vi "clear_selection_list.vi"(6 "wait for reply (T)":bool=TRUE, 8 "error in":errorcluster, 11 "vi_id":i32) -> (0 "error out":errorcluster, 1 "timed out?":bool)   [LabVIEW 2025, in "Scripting Server.lvlib"]
doc: "Clears all elements in the selection list. Use this before making a new selection.\n\n_____\nCreated using DQMH Framework: Event Scripter 7.1.0.1503."
uses:
  Scripting Server.lvlib
  clear_selection_list Argument--cluster.ctl
  clear_selection_list (Reply Payload)--cluster.ctl
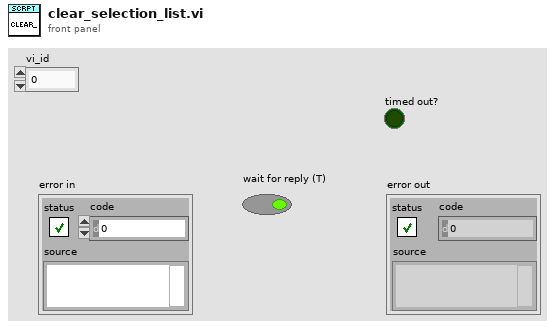
[diagram p1: front panel]
types:
  T1 = typedef "Scripting Server.lvlib/clear_selection_list Argument--cluster.ctl" = cluster{"Wait Notifier":refnum<notifier>, "wait for reply":bool, "vi_id":i32}
  T2 = typedef "Scripting Server.lvlib/Request Events--cluster.ctl" = cluster{"Stop Module":refnum<user-event>, "Show Panel":refnum<user-event>, "Hide Panel":refnum<user-event>, "Get Module Execution Status":refnum<user-event>, "Show Diagram":refnum<user-event>, "New VI":refnum<user-event>, "Add Object":refnum<user-event>, "Connect Objects":refnum<user-event>, "Get Object Terminals":refnum<user-event>, "get vi error list":refnum<user-event>, "Cleanup VI":refnum<user-event>, "create_control":refnum<user-event>, "Run VI":refnum<user-event>, "add_to_selection":refnum<user-event>, "clear_selection_list":refnum<user-event>, "remove_from_selection":refnum<user-event>, "enclose_selection":refnum<user-event>}
  T3 = typedef "Scripting Server.lvlib/clear_selection_list (Reply Payload)--cluster.ctl" = cluster{"error":errorcluster}
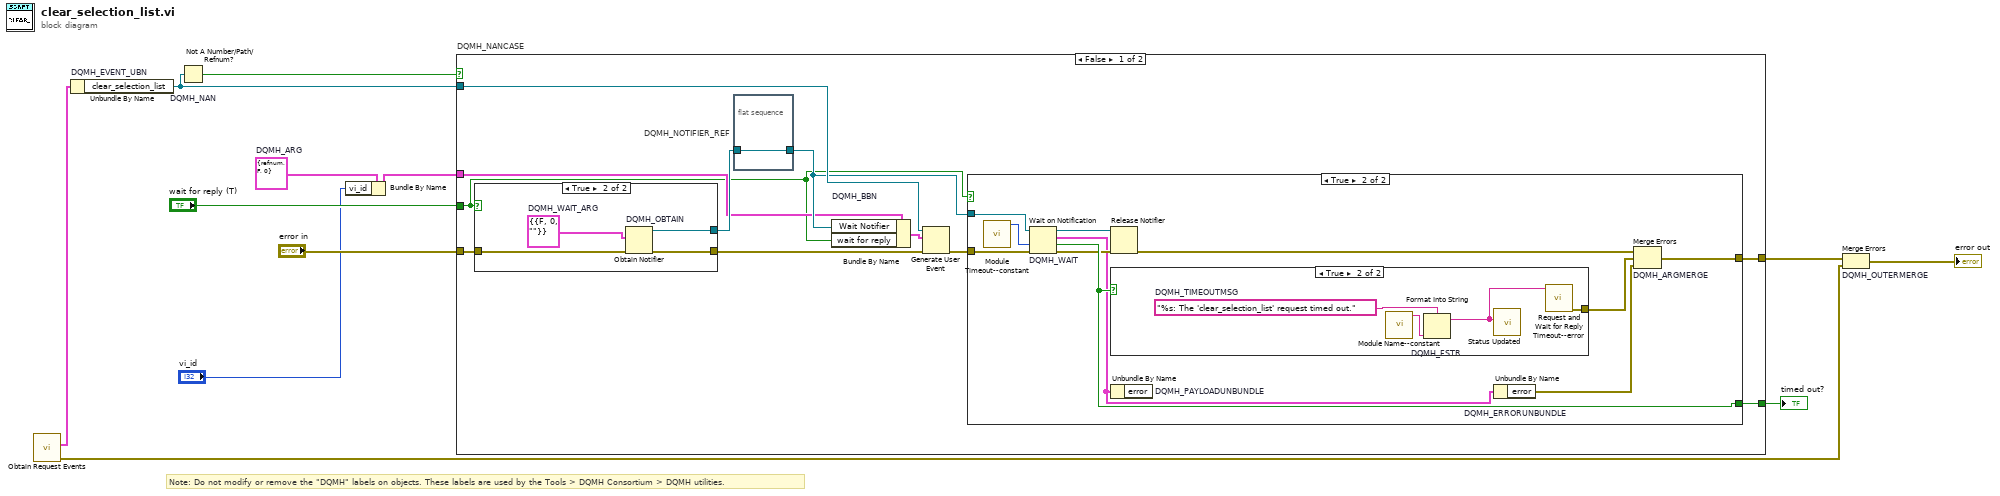
[diagram p0: block diagram]
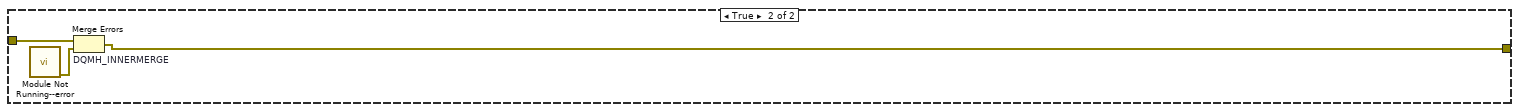
[diagram p5: hidden frame]
diagram:
  w6 = T1 {"Wait Notifier"=refnum, "wait for reply"=FALSE, "vi_id"=0}  # DQMH_ARG
  # "Note: Do not modify or remove the \"DQMH\" labels on objects. These labels are used by the Tools > DQMH Consortium > DQMH utilities."
  n1 = call "Obtain Request Events.vi"() -> ("error out"=w4:errorcluster, "Scripting Server Request Events"=w3:T2)  [unwired: 10 in]
  n2 = Unbundle By Name "DQMH_EVENT_UBN"(w3) -> ("clear_selection_list"=w10:refnum<user-event>)
  n3 = Not A Number/Path/Refnum? "DQMH_NAN"(number/path/refnum=w10) -> (NaN/Path/Refnum?=w9:bool)
  n4 = Bundle By Name(cluster=w6, "vi_id"="vi_id") -> (w2:T1)
  n5 = case "DQMH_NANCASE" shown="False" w9 {
    tunnel: "error in" -> [w23 w48]
    tunnel: w10 -> [w21 _]
    tunnel: [w18 w47] -> w7
    tunnel: [w19 _] -> w8
    tunnel: w2 -> [w14 _]
    tunnel: "wait for reply (T)" -> [w13 _]
    frame False {
      n6 = case shown="True" w13 {
        tunnel: w23 -> [w41 w45]
        tunnel: [w41 w44] -> w20
        tunnel: [_ w42] -> w16
        frame False {
        }
        frame True {
          w43 = T3 {"error"={"status"=FALSE, "code"=0, "source"=""}}  # DQMH_WAIT_ARG
          n7 = Obtain Notifier "DQMH_OBTAIN"(notification data type=w43, error in (no error)=w45) -> (notifier out=w42:refnum<notifier>, error out=w44:errorcluster)  [unwired: 2 in, 1 out]
        }
      }
      n8 = flat-sequence "DQMH_NOTIFIER_REF" {
        tunnel: w16 -> [w24]
        tunnel: [w24] -> w15
        frame #0 {
        }
      }
      n9 = Bundle By Name "DQMH_BBN"(cluster=w14, "Wait Notifier"=w15, "wait for reply"=w13) -> (w17:T1)
      n10 = Generate User Event(user event=w21, event data cluster=w17, error in=w20) -> (error out=w22:errorcluster)  [unwired: 1 in, 1 out]
      n11 = case shown="True" w13 {
        tunnel: w22 -> [w25 w36]
        tunnel: w15 -> [_ w35]
        tunnel: [_ w33] -> w19
        tunnel: [w25 w32] -> w18
        frame False {
        }
        frame True {
          n12 = call "Module Timeout--constant.vi"() -> ("Module Timeout"=w26:i32)  [unwired: 11 in]
          n13 = Wait on Notification "DQMH_WAIT"(notifier=w35, timeout in ms (-1)=w26, error in (no error)=w36) -> (notifier out=w34:refnum<notifier>, notification=w27:T3, timed out?=w33:bool, error out=w31:errorcluster)  [unwired: 1 in]
          n14 = Release Notifier(notifier=w34, error in (no error)=w31) -> (error out=w30:errorcluster)  [unwired: 1 in, 2 out]
          n15 = case shown="True" w33 {
            tunnel: [_ w38] -> w28
            frame False {
            }
            frame True {
              w40 = "%s: The 'clear_selection_list' request timed out."  # DQMH_TIMEOUTMSG
              n16 = call "Module Name--constant.vi"() -> ("Module Name"=w37:string)  [unwired: 11 in]
              n17 = Format Into String "DQMH_FSTR"(format string=w40, w37) -> (resulting string=w39:string)  [unwired: 2 in, 1 out]
              n18 = call "Status Updated.vi"("Status"=w39) -> ()  [unwired: 10 in, 1 out]
              n19 = call "Request and Wait for Reply Timeout--error.vi"("Error Message"=w39) -> ("error out"=w38:errorcluster)  [unwired: 10 in]
            }
          }
          n20 = Unbundle By Name "DQMH_PAYLOADUNBUNDLE"(w27) -> ()  [unwired: 1 out]
          n21 = Unbundle By Name "DQMH_ERRORUNBUNDLE"(w27) -> ("error"=w29:errorcluster)
          n22 = Merge Errors "DQMH_ARGMERGE"(w30, w28, w29) -> (w32:errorcluster)
        }
      }
    }
    frame True {
      n23 = call "Module Not Running--error.vi"() -> ("error out"=w46:errorcluster)  [unwired: 11 in]
      n24 = Merge Errors "DQMH_INNERMERGE"(w48, w46) -> (w47:errorcluster)
    }
  }
  "timed out?" <- w8
  n25 = Merge Errors "DQMH_OUTERMERGE"(w7, w4) -> (→"error out":errorcluster)
